vi "end of file.vi"(8 "error in (no error)":errorcluster, 10 "refnum out":refnum<file>, 11 "output cluster":T1={"DAQ Parameters"={"Sampling rate"=0.0, "Max_volt"=0.0, "Min_volt"=0.0, "DAQmx Physical Channels \nHR,SC"="", "Resting State"=FALSE, "Analyze every (s)"=0.01}, "Patient Info \n(Updates automatically when reading from file)"={"Patient Name"="", "Patient ID"="", "Patient Age"=0.0, "Gender"=""}, "Raw Data Read Path"=path "", "Avg HR "=0.0, "Avg SC  "=0.0} {"DAQ Parameters"."Analyze every (s)" min=0.01 max=10.0 step=0.01 scale=0.0..10.0; "DAQ Parameters"."Min_volt" min=-10.0 max=10.0 scale=-10.0..10.0; "DAQ Parameters"."Max_volt" min=-10.0 max=10.0 scale=-10.0..10.0}) -> (0 "error out":errorcluster)   [LabVIEW 2014]
uses:
  patiant and daq params.ctl
  set_get.ctl
  CMD DAQ enum.ctl
panel:
  # "Leave zero if unkown \nand run in Resting mode first"
  # "Active State"
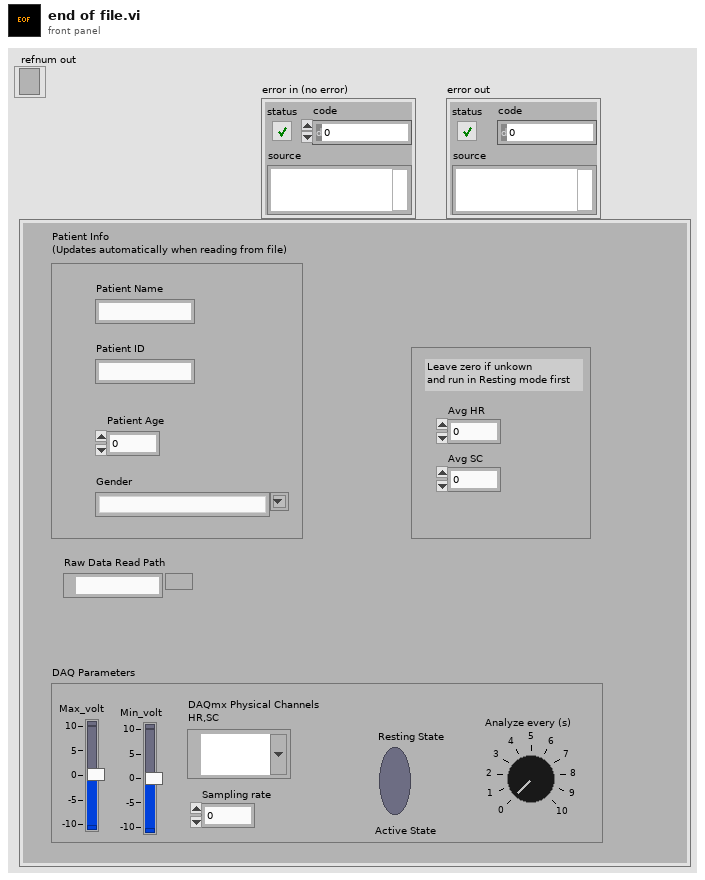
[diagram p1: front panel]
types:
  T1 = typedef "patiant and daq params.ctl" = cluster{"DAQ Parameters":cluster{"Sampling rate":dbl, "Max_volt":dbl, "Min_volt":dbl, "DAQmx Physical Channels \nHR,SC":tag, "Resting State":bool, "Analyze every (s)":dbl}, "Patient Info \n(Updates automatically when reading from file)":cluster{"Patient Name":string, "Patient ID":string, "Patient Age":dbl, "Gender":string}, "Raw Data Read Path":path, "Avg HR ":dbl, "Avg SC  ":dbl}
  T2 = typedef "CMD DAQ enum.ctl" = enum16{"Init DAQ", "Init Read From File", "DAQ", "Read From File", "Stop DAQ", "Stop Read From File", "Exit"}
  T3 = typedef "set_get.ctl" = enum16{"Set", "Get"}
  T4 = cluster{"CMD UI":refnum<queue>, "CMD REP":refnum<queue>, "CMD DA":refnum<queue>, "CMD DAQ":refnum<queue>, "CMD LOG":refnum<queue>, "Data LOG":refnum<queue>, "Data Display":refnum<queue>}
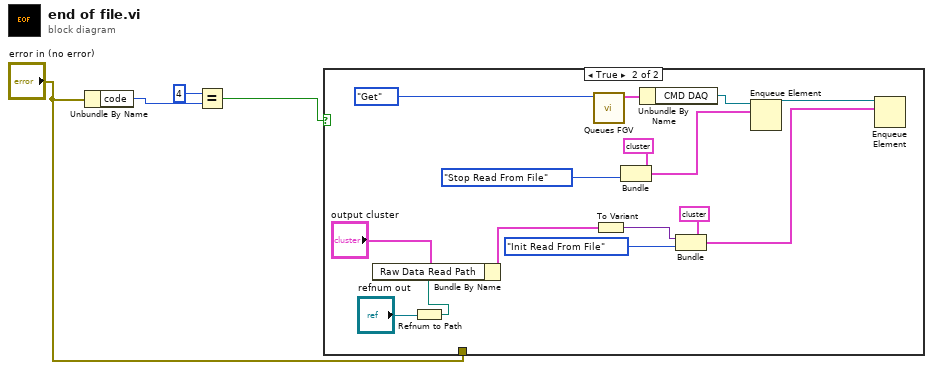
[diagram p0: block diagram]
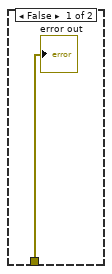
[diagram p2: hidden frame]
diagram:
  n1 = Unbundle By Name("error in (no error)") -> ("code"=w4:i32)
  n2 = Equal?(x=4, y=w4) -> (x = y?=w2:bool)
  n3 = case shown="True" w2 {
    tunnel: "error in (no error)" -> [w5 _]
    frame False {
      "error out" <- w5
    }
    frame True {
      n4 = Refnum to Path(1:"refnum out") -> (0:w8:path)
      n5 = Bundle By Name(cluster="output cluster", "Raw Data Read Path"=w8) -> (w7:T1)
      n6 = call "Queues FGV.vi"("Enum"=set_get."Get") -> ("Queues"=w16:T4)  [unwired: 10 in]
      n7 = To Variant(anything=w7) -> (Variant=w6:variant)
      n8 = Bundle(cluster=cluster{variant, T2} {variant, enum."Init DAQ"}, CMD_DAQ_enum."Stop Read From File") -> (w20:cluster{variant, T2})  [unwired: 1 in]
      n9 = Unbundle By Name(w16) -> ("CMD DAQ"=w17:refnum<queue>)
      n10 = Bundle(cluster=cluster{variant, T2} {variant, enum."Init DAQ"}, w6, CMD_DAQ_enum."Init Read From File") -> (w11:cluster{variant, T2})
      n11 = Enqueue Element(queue=w17, element=w20) -> (queue out=w14:refnum<queue>)  [unwired: 2 in, 2 out]
      n12 = Enqueue Element(queue=w14, element=w11) -> ()  [unwired: 2 in, 3 out]
    }
  }
